vi "Initialize Camera.vi"(8 "error in (no error)":errorcluster, 10 "channel":u16, 11 "CCDCamera in":refnum<class "Simulated_CCD_Camera.lvclass">) -> (0 "error out":errorcluster, 3 "CCDCamera out":refnum<class "Simulated_CCD_Camera.lvclass">)   [LabVIEW 2018, in "Simulated_CCD_Camera.lvclass"]
uses:
  Simulated_CCD_Camera.lvclass
  Simulated_CCD_Camera.lvclass/Simulated_CCD_Camera.ctl
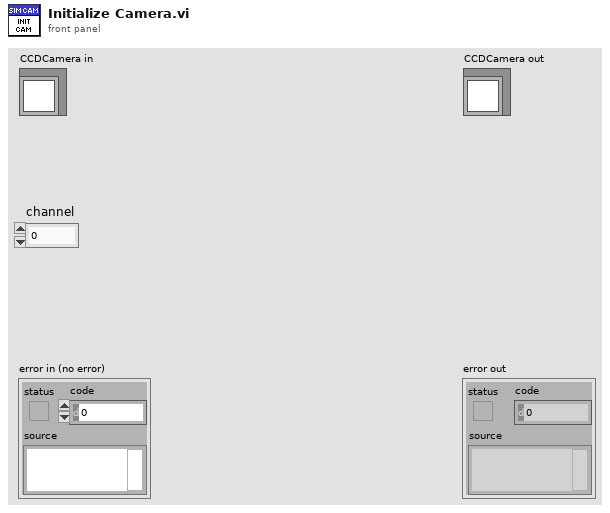
[diagram p1: front panel]
types:
  T1 = cluster{"CUBE_EXPOSURE_TIME":sgl, "CUBES_DONE":u16, "LAST_IMAGE_NAME":string, "DISK_SPACE":u16, "FRAMES_DONE":u16, "CCD_STATUS":string, "CURRENT_TEMPERATURE":i16, "TEMPERATURE_STATUS":string, "FRAME_EXPOSURE_TIME":sgl, "CCD_POWER_STATUS":bool, "SERIAL_NUMBER":u16, "ACQUIRING":bool}
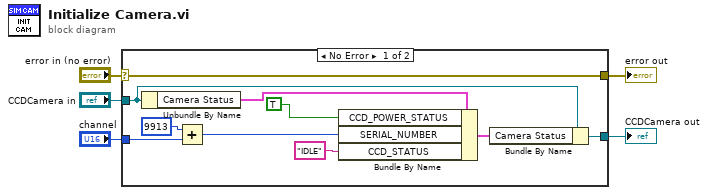
[diagram p0: block diagram]
diagram:
  n1 = case shown="No Error" "error in (no error)" {
    selector: "error in (no error)" -> [w15 w17]
    tunnel: [w15 w17] -> w2
    tunnel: [w12 w16] -> w3
    tunnel: "CCDCamera in" -> [w11 w16]
    tunnel: "channel" -> [w8 _]
    frame No Error {
      n2 = Unbundle By Name(w11) -> ("Camera Status"=w7:T1)
      n3 = Add(x=u16 9913 ("Initialization.Serial Number"), y=w8) -> (x+y=w9:u16)
      n4 = Bundle By Name(cluster=w7, "CCD_POWER_STATUS"=TRUE ("Initialization"), "SERIAL_NUMBER"=w9, "CCD_STATUS"="IDLE" ("Camera Status.STATUS")) -> (w6:T1)
      n5 = Bundle By Name(cluster=w11, "Camera Status"=w6) -> (w12:refnum<class "Simulated_CCD_Camera.lvclass">)
    }
    frame Error {
    }
  }
  "error out" <- w2
  "CCDCamera out" <- w3
